vi "users.vi"(7 "httpRequestID":u32) -> ()   [LabVIEW 2011]
doc: "This VI is a state machine that can be ran from a Browser."
uses:
  server/database/Users/User Record.ctl
  <vilib>/addons/internet/utils/strutil.llb/Case Matching.ctl
  <vilib>/wsapi/NI_WebServices.lvlib
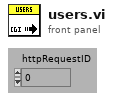
[diagram p1: front panel]
types:
  T1 = typedef "User Record.ctl" = cluster{"ixUser":i32, "sxUsername":string, "sLastName":string, "sFirstName":string, "sEmail":string, "sPassword":string, "tLoginTime":timestamp, "sLoginComputer":string, "fAdministrator":bool, "fRunSequences":bool, "fModifySequences":bool, "fRunScenarios":bool, "fModifyScenarios":bool, "fModifyTemplates":bool, "fModifyUsers":bool, "fModifyStations":bool, "fModifyFields":bool}
  T2 = typedef "Connection Refnum.ctl" = cluster{"Environment Handle":i32, "Connection Handle":i32}
  T3 = typedef "Case Matching.ctl" = enum16{"a != A", "a == A", "system"}
  T4 = typedef "Keyed Array.ctl" = cluster{"keys":string[], "values":string[]}
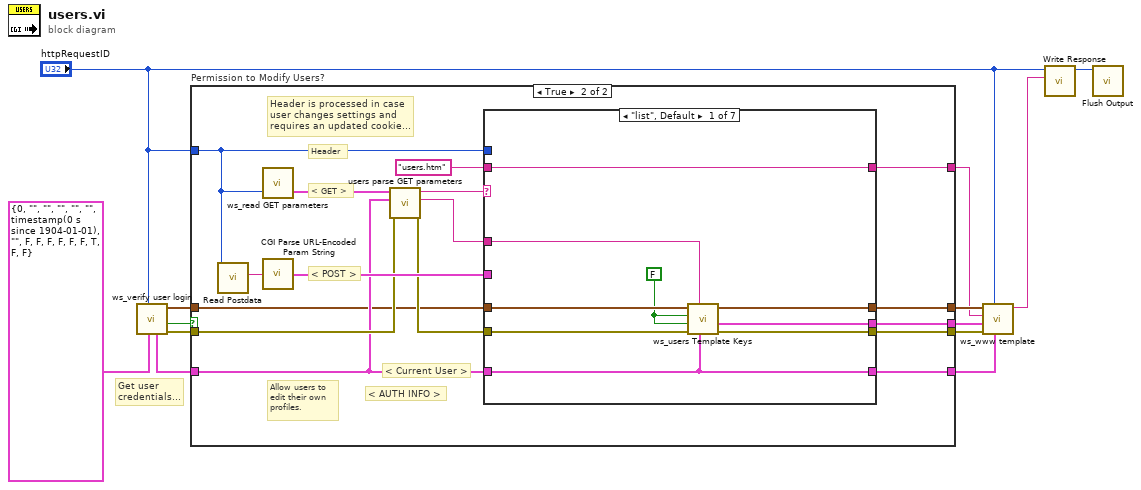
[diagram p0: block diagram]
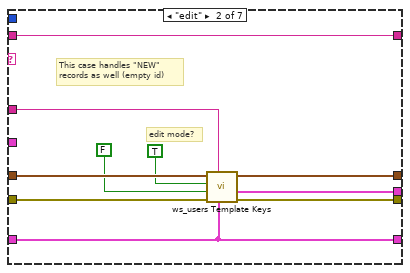
[diagram p3: hidden frame]
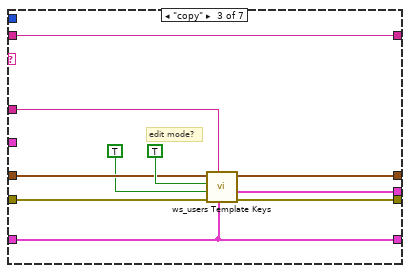
[diagram p4: hidden frame]
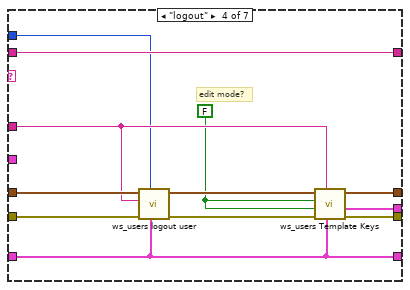
[diagram p5: hidden frame]
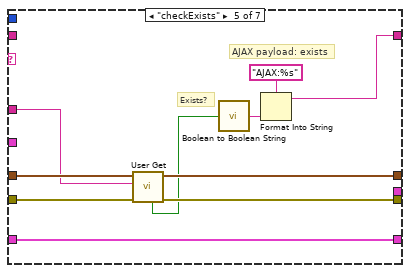
[diagram p6: hidden frame]
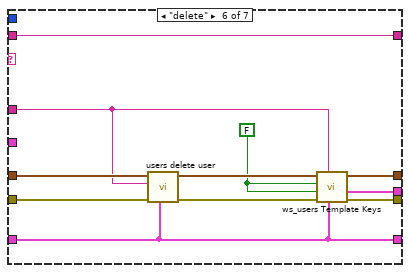
[diagram p7: hidden frame]
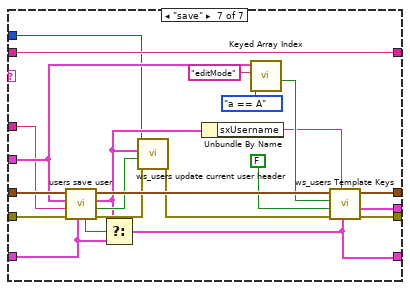
[diagram p8: hidden frame]
diagram:
  # "Get user \ncredentials..."
  n1 = call "ws_verify user login.vi"("Required Permisions"=T1 {"ixUser"=0, "sxUsername"="", "sLastName"="", "sFirstName"="", "sEmail"="", "sPassword"="", "tLoginTime"=timestamp(0 s since 1904-01-01), "sLoginComputer"="", "fAdministrator"=FALSE, "fRunSequences"=FALSE, "fModifySequences"=FALSE, "fRunScenarios"=FALSE, "fModifyScenarios"=FALSE, "fModifyTemplates"=FALSE, "fModifyUsers"=TRUE, "fModifyStations"=FALSE, "fModifyFields"=FALSE}, "httpRequestID"="httpRequestID") -> ("error out"=w6:errorcluster, "User Verified\nand Spartan\nAuthorized?"=w5:bool, "DB Connection Ref"=w4:T2, "User"=w3:T1)  [unwired: 6 in]
  n2 = case "Permission to Modify Users?" shown="True" w5 {
    tunnel: w3 -> [w14 w28]
    tunnel: w4 -> [w15 w19]
    tunnel: w6 -> [w16 w31]
    tunnel: [w16 w26] -> w12
    tunnel: [w15 w25] -> w13
    tunnel: [_ w23] -> w9
    tunnel: [w14 w21] -> w10
    tunnel: [_ w24] -> w11
    tunnel: "httpRequestID" -> [_ w17]
    frame False {
    }
    frame True {
      # "< AUTH INFO >"
      # "Allow users to\nedit their own\nprofiles."
      # "< GET >"
      # "< Current User >"
      # "Header is processed in case\nuser changes settings and\nrequires an updated cookie..."
      # "Header"
      # "< POST >"
      n3 = call <vilib>:"Read Postdata.vi"("httpRequestID"=w17) -> ("postdata"=w18:string)  [unwired: 8 in, 2 out]
      n4 = call "ws_read GET parameters.vi"("httpRequestID"=w17) -> ("GET query params"=w22:T4)  [unwired: 2 in]
      n5 = call <vilib>:"CGI Parse URL-Encoded Param String.vi"("url-encoded param string"=w18) -> ("params"=w32:T4)
      n6 = call "users parse GET parameters.vi"("error in (no error)"=w31, "Current User (none)"=w28, "GET (empty)"=w22) -> ("error out"=w20:errorcluster, "Parameter"=w29:string, "Command"=w30:string)  [unwired: 6 out]
      n7 = case shown="\"list\", Default" w30 {
        tunnel: [w40 w50 w60 w72 w81 w89 w109] -> w26
        tunnel: [w39 w49 w58 w71 w80 w91 w110] -> w25
        tunnel: w20 -> [w36 w46 w55 w69 w78 w94 w116]
        tunnel: w19 -> [w37 w47 w56 w68 w82 w93 w115]
        tunnel: w29 -> [w34 w44 w53 w64 w76 w85 w99]
        tunnel: w32 -> [_ _ _ _ _ _ w114]
        tunnel: w28 -> [w35 w45 w54 w65 w77 w86 w101]
        tunnel: "users.htm" ("Template (\"\")") -> [w41 w51 w61 w73 _ w87 w107]
        tunnel: [w41 w51 w61 w73 w79 w87 w107] -> w23
        tunnel: [w38 w48 w57 w70 _ w88 w108] -> w24
        tunnel: [w35 w45 w54 w65 w77 w86 w98] -> w21
        tunnel: w17 -> [_ _ _ w62 _ _ w95]
        frame "list", Default {
          w33 = FALSE
          n8 = call "ws_users Template Keys.vi"("Current User Record"=w35, "Edit sxUsername (\"\")"=w34, "error in (no error)"=w36, "Copy? (f)"=w33, "Edit? (f)"=w33, "Connection Refnum"=w37) -> ("error out"=w40:errorcluster, "Template Keys"=w38:T4, "Connection Refnum"=w39:T2)  [unwired: 1 in, 2 out]
        }
        frame "edit" {
          # "This case handles \"NEW\"\nrecords as well (empty id)"
          # "edit mode?"
          n9 = call "ws_users Template Keys.vi"("Current User Record"=w45, "Edit sxUsername (\"\")"=w44, "error in (no error)"=w46, "Copy? (f)"=FALSE, "Edit? (f)"=TRUE, "Connection Refnum"=w47) -> ("error out"=w50:errorcluster, "Template Keys"=w48:T4, "Connection Refnum"=w49:T2)  [unwired: 1 in, 2 out]
        }
        frame "copy" {
          # "edit mode?"
          n10 = call "ws_users Template Keys.vi"("Current User Record"=w54, "Edit sxUsername (\"\")"=w53, "error in (no error)"=w55, "Copy? (f)"=TRUE, "Edit? (f)"=TRUE, "Connection Refnum"=w56) -> ("error out"=w60:errorcluster, "Template Keys"=w57:T4, "Connection Refnum"=w58:T2)  [unwired: 1 in, 2 out]
        }
        frame "logout" {
          w63 = FALSE
          # "edit mode?"
          n11 = call "ws_users logout user.vi"("Current User"=w65, "httpRequestID"=w62, "error in (no error)"=w69, "Username to Logout (\"\")"=w64, "Connection Refnum"=w68) -> ("error out"=w66:errorcluster, "Connection Refnum"=w67:T2)  [unwired: 5 in]
          n12 = call "ws_users Template Keys.vi"("Current User Record"=w65, "Edit sxUsername (\"\")"=w64, "error in (no error)"=w66, "Copy? (f)"=w63, "Edit? (f)"=w63, "Connection Refnum"=w67) -> ("error out"=w72:errorcluster, "Template Keys"=w70:T4, "Connection Refnum"=w71:T2)  [unwired: 1 in, 2 out]
        }
        frame "checkExists" {
          # "AJAX payload: exists"
          # "Exists?"
          n13 = call "User Get.vi"("error in (no error)"=w78, "sxUsername (\"\")"=w76, "Connection Refnum"=w82) -> ("error out"=w81:errorcluster, "Connection Refnum"=w80:T2, "Data Present?"=w75:bool)  [unwired: 6 out]
          n14 = call "Boolean to Boolean String.vi"("Boolean"=w75) -> ("Boolean string"=w74:string)  [unwired: 1 in]
          n15 = Format Into String(format string="AJAX:%s", w74) -> (resulting string=w79:string)  [unwired: 2 in, 1 out]
        }
        frame "delete" {
          w84 = FALSE
          n16 = call "users delete user.vi"("Current User (none)"=w86, "error in (no error)"=w94, "Username (\"\")"=w85, "Connection Refnum"=w93) -> ("error out"=w90:errorcluster, "Connection Refnum"=w92:T2)  [unwired: 6 out]
          n17 = call "ws_users Template Keys.vi"("Current User Record"=w86, "Edit sxUsername (\"\")"=w85, "error in (no error)"=w90, "Copy? (f)"=w84, "Edit? (f)"=w84, "Connection Refnum"=w92) -> ("error out"=w89:errorcluster, "Template Keys"=w88:T4, "Connection Refnum"=w91:T2)  [unwired: 1 in, 2 out]
        }
        frame "save" {
          n18 = call "users save user.vi"("Current User"=w101, "error in (no error)"=w116, "Username (\"\")"=w99, "POST (empty)"=w114, "Connection Ref"=w115) -> ("error out"=w105:errorcluster, "User Credentials Change?"=w103:bool, "new User Record"=w96:T1, "dup Connection Ref"=w111:T2, "Current Record Edit?"=w102:bool)  [unwired: 2 in]
          n19 = Select(t=w96, s=w102, f=w101) -> (s? t:f=w98:T1)
          n20 = call "ws_users update current user header.vi"("error in (no error)"=w105, "Current User Changes? (f)"=w103, "new Current User"=w96, "httpRequestID"=w95) -> ("error out"=w104:errorcluster)  [unwired: 7 in]
          n21 = Unbundle By Name(w96) -> ("sxUsername"=w97:string)
          n22 = call <vilib>:"Keyed Array Index.vi"("case matching (sensitive)"=Case_Matching."a == A", "key"="editMode", "array in"=w114) -> ("valid key"=w106:bool)  [unwired: 1 in, 3 out]
          n23 = call "ws_users Template Keys.vi"("Current User Record"=w98, "Edit sxUsername (\"\")"=w97, "error in (no error)"=w104, "Copy? (f)"=FALSE, "Edit? (f)"=w106, "Connection Refnum"=w111) -> ("error out"=w109:errorcluster, "Template Keys"=w108:T4, "Connection Refnum"=w110:T2)  [unwired: 1 in, 2 out]
        }
      }
    }
  }
  n24 = call "ws_www template.vi"("User"=w10, "httpRequestID"="httpRequestID", "error in (no error)"=w12, "Template Keys (empty)"=w11, "Template (\"\")"=w9, "DB Connection Ref"=w13) -> ("HTTP Template Content"=w8:string)  [unwired: 5 in]
  n25 = call <vilib>:"Write Response.vi"("response string"=w8, "httpRequestID"="httpRequestID") -> ("httpRequestID out"=w7:u32)  [unwired: 8 in, 1 out]
  n26 = call <vilib>:"Flush Output.vi"("httpRequestID"=w7) -> ()  [unwired: 9 in, 2 out]
